vi "String To Date.vi"(8 "error in (no error)":errorcluster, 11 "String to Convert":string) -> (0 "error out":errorcluster, 3 "Date Value":timestamp format="%<%x>T")   [LabVIEW 2023, in "HAF.lvlib"]
doc: "Converts the passed String Value to a Date only timestamp - the time portion is set to midnight. The passed string must be in the format defined by the system, e.g. DD/MM/YYYY, otherwise an invalid conversion may be returned. Day and month can be single digits, year must be 4 digits."
uses:
  HAF.lvlib
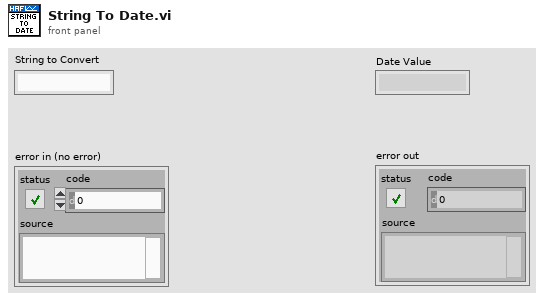
[diagram p1: front panel]
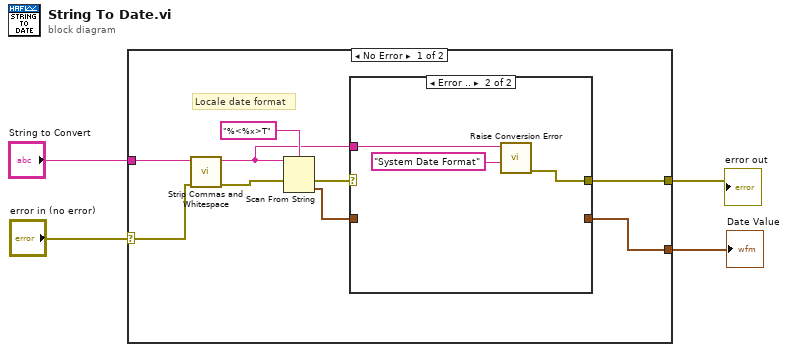
[diagram p0: block diagram]
diagram:
  n1 = case shown="No Error" "error in (no error)" {
    selector: "error in (no error)" -> [w12 w19]
    tunnel: "String to Convert" -> [w13 _]
    tunnel: [w6 w19] -> w2
    tunnel: [w5 _] -> w1
    frame No Error {
      # "Locale date format"
      n2 = call "Strip Commas and Whitespace.vi"("error in (no error)"=w12, "String to Strip"=w13) -> ("error out"=w11:errorcluster, "Clean String"=w9:string)  [unwired: 8 in]
      n3 = Scan From String(format string="%<%x>T", input string=w9, error in=w11) -> (error out=w8:errorcluster, output 1=w7:timestamp)  [unwired: 2 in, 2 out]
      n4 = case shown="Error .." w8 {
        selector: w8 -> [w15 _]
        tunnel: w9 -> [_ w18]
        tunnel: w7 -> [w14 _]
        tunnel: [w15 w16] -> w6
        tunnel: [w14 _] -> w5
        frame No Error {
        }
        frame Error {
          n5 = call "Raise Conversion Error.vi"("Data Type Attempted"="System Date Format", "String in Error"=w18) -> ("error out"=w16:errorcluster)  [unwired: 9 in]
        }
      }
    }
    frame Error {
    }
  }
  "Date Value" <- w1
  "error out" <- w2
